vi "ExposeListen.vi"(8 "error in (no error)":errorcluster, 11 "Expose Info":T1) -> (0 "error out":errorcluster)   [LabVIEW 2017]
uses:
  ExposeInfo.ctl
  C:/Code/CMCryoSysCode/Expose/COM/CSCom/CSCom/bin/Release/CSCom.dll
  COM/CSCom/CSCom/bin/Release/CSCom.dll
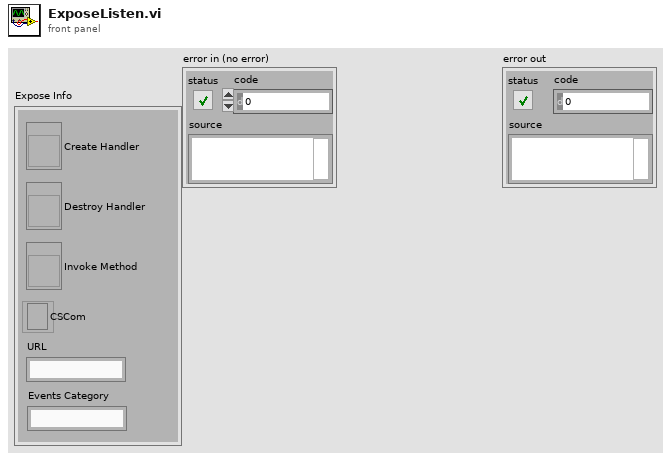
[diagram p1: front panel]
types:
  T1 = typedef "ExposeInfo.ctl" = cluster{"Create Handler":refnum<vi>, "Destroy Handler":refnum<vi>, "Invoke Method":refnum<vi>, "CSCom":refnum<k24>, "URL":string, "Events Category":string}
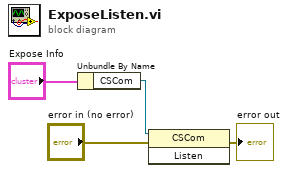
[diagram p0: block diagram]
diagram:
  n1 = Unbundle By Name("Expose Info") -> ("CSCom"=w3:refnum<k24>)
  n2 = invoke class="CSCom" method="Listen"(reference=w3, error in="error in (no error)") -> (error out=→"error out":errorcluster)  [unwired: 1 in, 2 out]
